vi "UDP.Rx.Top.vi"(8 "error in (no error)":errorcluster, 9 "max size (800)":i32=800, 10 "ports":u16[](array[numeric])=[60000, 60001, 60002, 60003], 11 "Stop Pointer":refnum<class "Memory.Pointer.lvclass">) -> (0 "error out":errorcluster)   [LabVIEW 2017]
uses:
  <vilib>/National Instruments/Memory Manager/Classes/Pointer/Memory.Pointer.lvclass
  <vilib>/National Instruments/Memory Manager/Classes/Pointer/Memory.Pointer.lvclass/Memory.Pointer.ctl
  <vilib>/National Instruments/Memory Manager/Classes/Pointer/Memory.Pointer.Read.0D.I32.vi
  <vilib>/National Instruments/Memory Manager/Classes/Pointer/Memory.Pointer.Write.0D.Bool.vi
  <vilib>/National Instruments/Memory Manager/Classes/Pointer/Memory.Pointer.Read.0D.Bool.vi
  <vilib>/National Instruments/Memory Manager/Classes/Pointer/Memory.Pointer.Read.No Check.0D.I32.vi
  <vilib>/National Instruments/Memory Manager/Classes/Pointer/Memory.Pointer.Parameter Check.Null Pointer.vi
  <vilib>/National Instruments/Memory Manager/Classes/Pointer/Memory.Pointer.Parameter Check.Subset.vi
  <vilib>/National Instruments/Memory Manager/Classes/Pointer/Memory.Pointer.Write.No Check.0D.Bool.vi
  <vilib>/National Instruments/Memory Manager/Classes/Pointer/Memory.Pointer.Read.No Check.0D.Bool.vi
  <vilib>/National Instruments/Memory Manager/Classes/Pointer/Memory.Pointer.Get Address.vi
  <vilib>/National Instruments/Memory Manager/Classes/Pointer/Memory.Pointer.Errors.vi
  <vilib>/National Instruments/Memory Manager/Classes/Pointer/Memory.Pointer.Errors.Null Pointer.vi
  <vilib>/National Instruments/Memory Manager/Classes/Pointer/Memory.Pointer.Errors.Out of Bounds.vi
  <vilib>/National Instruments/Memory Manager/Classes/Pointer/Memory.Pointer.Get Size.vi
  <vilib>/National Instruments/Memory Manager/Classes/Pointer/Memory.Pointer.Errors.Create Error.vi
  <vilib>/NI/Static Error Handling/VIs/Static Error Handling.Source Buffer.Write.String.vi
  <vilib>/National Instruments/Memory Manager/Classes/Pointer/Memory.Pointer.Errors.Write Pointer Size.vi
  <vilib>/NI/Static Error Handling/VIs/Static Error Handling.Source Buffer.Write.Numeric.Scalar.Base10.vi
  <vilib>/NI/Static Error Handling/VIs/Static Error Handling.Source Buffer.Write.Numeric.Scalar.Base10 (U64).vi
  <vilib>/NI/Static Error Handling/VIs/Static Error Handling.Error Cluster Constant.vi
  <vilib>/NI/Static Error Handling/VIs/Static Error Handling.Error Cluster Constant (512B).vi
  <vilib>/NI/Static Error Handling/VIs/Static Error Handling.Parameters.Status.Set.vi
  <vilib>/NI/Static Error Handling/VIs/Static Error Handling.Parameters.Code.Set.vi
  <vilib>/NI/Static Error Handling/VIs/Static Error Handling.Parameters.VI Source.Set.vi
  <vilib>/National Instruments/Memory Manager/Constants/Memory.Constants.vi
  <vilib>/National Instruments/Memory Manager/Constants/Memory.Constants.Library Name.vi
  <vilib>/National Instruments/Memory Manager/Classes/Pointer/Memory.Pointer.Errors.Get Info.vi
panel:
  in  "Stop 2":bool
  out "rx counts":i32[](array[numeric])
  in  "Stop":bool
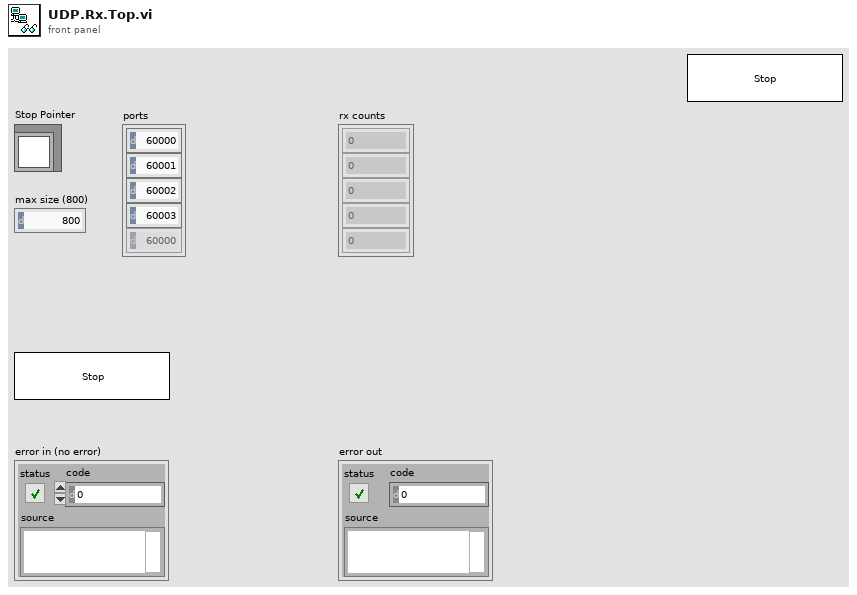
[diagram p1: front panel]
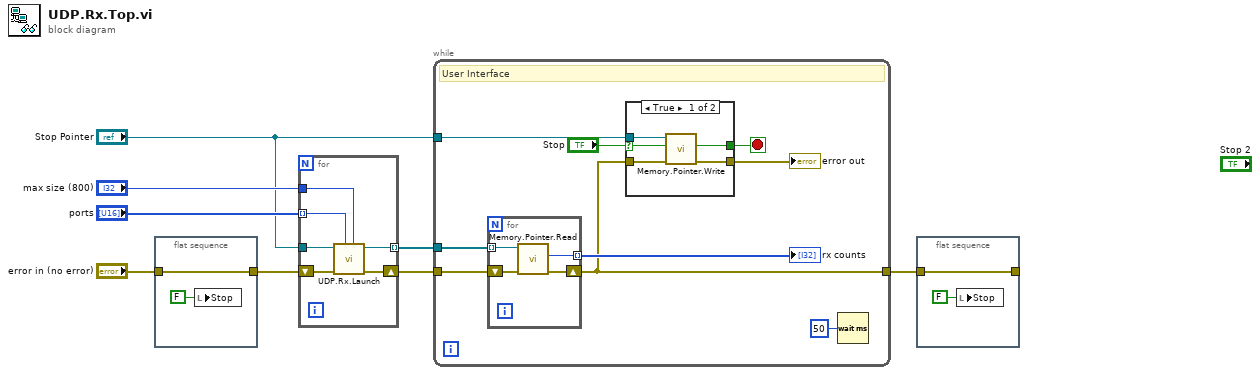
[diagram p0: block diagram]
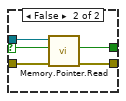
[diagram p2: hidden frame]
diagram:
  n1 = flat-sequence {
    tunnel: "error in (no error)" -> [w10]
    tunnel: [w10] -> w2
    frame #0 {
      n2 = local write "Stop"(FALSE ("Stop")) -> ()
    }
  }
  n3 = for {
    tunnel: "Stop Pointer" -> [w11]
    tunnel: "ports" -> [w14] mode=indexing
    tunnel: "max size (800)" -> [w13]
    shift-right: [w16] -> w6
    shift-left: w2 -> [w15]
    tunnel: [w12] -> w5 mode=indexing
    n4 = call "UDP.Rx.Launch.vi"("max size (548)"=w13, "port"=w14, "error in (no error)"=w15, "Stop Pointer"=w11) -> ("error out"=w16:errorcluster, "Count Pointer"=w12:refnum<class "Memory.Pointer.lvclass">)  [unwired: 6 in]
  }
  n5 = while {
    tunnel: w6 -> [w24]
    tunnel: w5 -> [w25]
    tunnel: "Stop Pointer" -> [w23]
    tunnel: [w17] -> w1
    stop <- w22 stop-if-true
    # "User Interface"
    n6 = for {
      tunnel: w25 -> [w39] mode=indexing
      tunnel: [w37] -> w19 mode=indexing
      shift-right: [w36] -> w17
      shift-left: w24 -> [w38]
      n7 = call-poly <vilib>:"Memory.Pointer.Read.vi"("error in (no error)"=w38, "Pointer in"=w39) -> ("error out"=w36:errorcluster, "value out"=w37:i32)  [unwired: 6 in, 2 out]
    }
    "rx counts" <- w19
    n8 = case shown="True" "Stop" {
      selector: "Stop" -> [w26 w31]
      tunnel: w23 -> [w30 w35]
      tunnel: w17 -> [w29 w34]
      tunnel: [w28 w33] -> w22
      tunnel: [w27 w32] -> w20
      frame True {
        n9 = call-poly <vilib>:"Memory.Pointer.Write.vi"("error in (no error)"=w29, "value"=w26, "Pointer in"=w30) -> ("error out"=w27:errorcluster, "value"=w28:bool)  [unwired: 5 in, 2 out]
      }
      frame False {
        n10 = call-poly <vilib>:"Memory.Pointer.Read.vi"("error in (no error)"=w34, "value in"=w31, "Pointer in"=w35) -> ("error out"=w32:errorcluster, "value out"=w33:bool)  [unwired: 5 in, 2 out]
      }
    }
    "error out" <- w20
    n11 = Wait (ms)(milliseconds to wait=u32 50) -> ()  [unwired: 1 out]
  }
  n12 = flat-sequence {
    tunnel: w1 -> [w41]
    tunnel: [w41] -> _
    frame #0 {
      n13 = local write "Stop"(FALSE ("Stop")) -> ()
    }
  }
